vi "scanclass_10ms_1dt.vi"() -> (0 "max jitter (uS)":dbl format="%.2f", 1 "mean time (uS)":dbl format="%.2f", 2 "standard deviation (uS)":dbl format="%.2f", 3 "execution histogram":T1(graph), 4 "Error":errorcluster, 5 "execution times (uS)":dbl[](graph))   [LabVIEW 2013]
uses:
  <vilib>/platform/TimedLoop/XDataNode/XDataNode.xnode
  <vilib>/Platform/TimedLoop/XDataNode/nitl_modes.ctl
  <vilib>/Platform/TimedLoop/XDataNode/XDNodeRunTimeDep.lvlib
  <vilib>/Platform/TimedLoop/XDataNode/wakeup.ctl
  <vilib>/Platform/TimedLoop/XDataNode/timing_clust.ctl
  scan engine timing source/scan engine timing source.lvclass
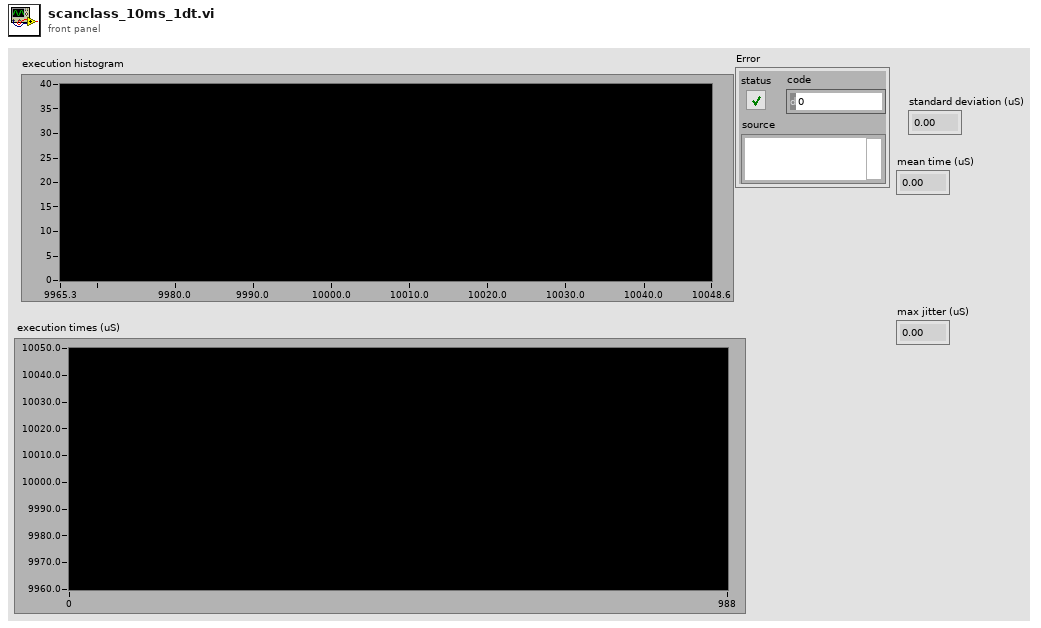
[diagram p1: front panel]
types:
  T1 = cluster{"X Values":dbl[], "Histogram: h(x)":i32[]}
  T2 = typedef "XDNodeRunTimeDep.lvlib/timing_clust.ctl" = cluster{"Expected End [f-1]":u64, "Actual End [f-1]":u64, "Finished Late? [f-1]":bool, "Expected End [i-1]":u64, "Actual End [i-1]":u64, "Finished Late? [i-1]":bool, "Expected Start [i]":u64, "Actual Start [i]":u64, "Expected Start [f]":u64, "Actual Start [f]":u64, "Source Name":string, "Structure Name":string, "Period":i64, "Deadline":i64, "Offset":i64, "Start":i64, "Priority":i32, "Timeout":i32, "Mode":T3, "Wakeup Reason":T4, "Error":errorcluster, "Source Type":string, "Secondary Source Type":string, "Global End Time":u64, "Global Start Time":u64, "Frame Duration":u64, "Iteration Duration":u64, "Assigned CPU":i32, "I/O Scan Engine Mode":u32}
  T3 = typedef "XDNodeRunTimeDep.lvlib/nitl_modes.ctl" = enum32{"No Change", "Process missed periods, maintain original phase", "Discard missed periods, maintain original phase", "Process missed periods, ignore original phase", "Discard missed periods, ignore original phase"}
  T4 = typedef "XDNodeRunTimeDep.lvlib/wakeup.ctl" = enum32{"Normal", "Aborted", "Asynchronous wakeup", "Timing source error", "Timed loop error", "Timeout"}
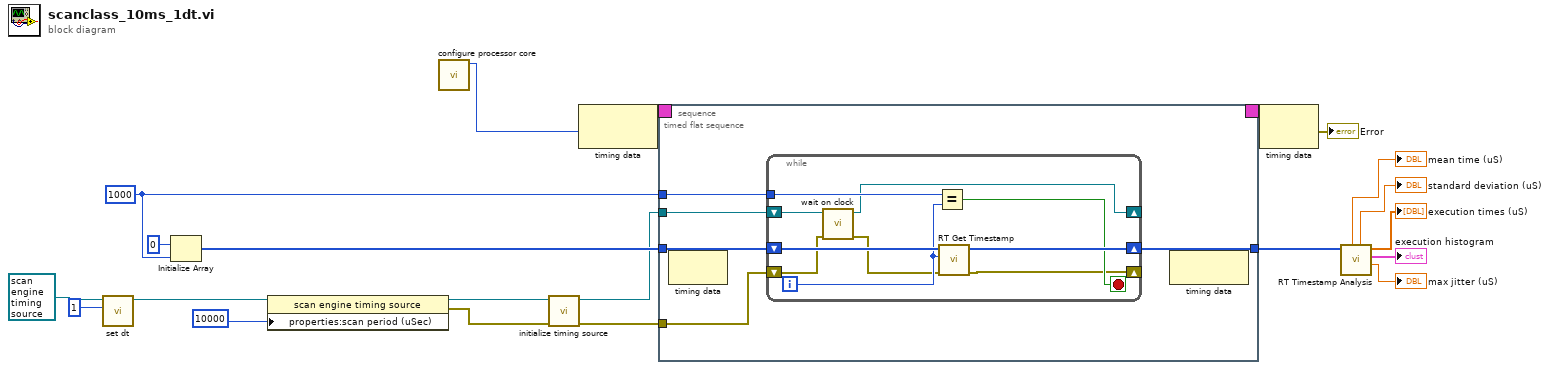
[diagram p0: block diagram]
diagram:
  w19 = 1000 ("x")
  n1 = call "set dt.vi"("dt"=u16 1, "timing source in"=refnum<class "scan engine timing source.lvclass"> refnum ("scan engine timing source.lvclass")) -> ("timing source out"=w6:refnum<class "scan engine timing source.lvclass">)  [unwired: 9 in]
  n2 = Initialize Array(u64 0, w19) -> (w20:u64[])
  n3 = property class="scan engine timing source"(reference=w6, "properties:scan period (uSec)"=u32 10000 ("scan period (uSec)")) -> (reference out=w4:refnum<class "scan engine timing source.lvclass">, error out=w2:errorcluster)  [unwired: 1 in]
  n4 = call "configure processor core.vi"() -> ("Processor"=w7:i32)  [unwired: 11 in]
  n5 = call-dynamic "initialize timing source.vi"("error in"=w2, "timing source in"=w4) -> ("error out"=w1:errorcluster, "timing source out"=w5:refnum<class "scan engine timing source.lvclass">)  [unwired: 8 in]
  n6 = node-c288(w7) -> (w12:T2)
  n7 = timed-sequence {
    timing: w12 -> [_]
    timing-out: [_] -> w11
    tunnel: w19 -> [w26]
    tunnel: w20 -> [w25]
    tunnel: [w24] -> w18
    tunnel: w5 -> [w23]
    tunnel: w1 -> [w22]
    n8 = timed-flat-sequence {
      tunnel: w26 -> [w31]
      tunnel: w25 -> [w30]
      tunnel: [w29] -> w24
      tunnel: w23 -> [w28]
      tunnel: w22 -> [w27]
      n9 = node-c288() -> ()  [unwired: 1 in, 1 out]
      n10 = while {
        tunnel: w31 -> [w41]
        shift-right: [w39] -> w29
        shift-left: w30 -> [w40]
        shift-right: [w34] -> _
        shift-left: w28 -> [w35]
        shift-right: [w33] -> _
        shift-left: w27 -> [w32]
        i -> [w37]
        stop <- w38 stop-if-true
        n11 = call-dynamic "wait on clock.vi"("error in"=w32, "timing source in"=w35) -> ("error out"=w36:errorcluster, "timing source out"=w34:refnum<class "scan engine timing source.lvclass">)  [unwired: 7 in, 1 out]
        n12 = Equal?(x=w41, y=w37) -> (x = y?=w38:bool)
        n13 = call <vilib>:"RT Get Timestamp.vi"("error in (no error)"=w36, "iteration"=w37, "timestamp array in"=w40) -> ("error out"=w33:errorcluster, "timestamp array out"=w39:u64[])  [unwired: 7 in]
      }
      n14 = node-c288() -> ()  [unwired: 1 in, 1 out]
    }
  }
  n15 = node-c288(w11) -> (→"Error":errorcluster)
  n16 = call <vilib>:"RT Timestamp Analysis.vi"("timestamp array"=w18) -> ("max jitter (uS)"=→"max jitter (uS)":dbl, "execution histogram"=→"execution histogram":T1, "execution times (uS)"=→"execution times (uS)":dbl[], "standard deviation (uS)"=→"standard deviation (uS)":dbl, "mean time (uS)"=→"mean time (uS)":dbl)  [unwired: 5 in, 1 out]
